vi "Build Qualified Class Private Data Name.vi"(1 "Qualified LabVIEW Class Name":string[](array[string])) -> (0 "Qualified LabVIEW Class Private Data Name":string)   [LabVIEW 2020]
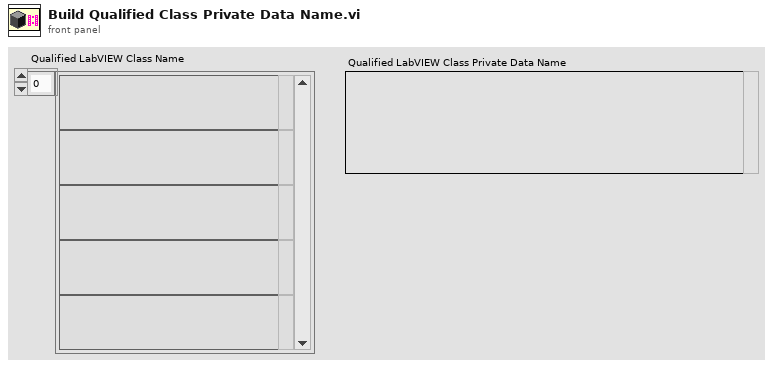
[diagram p1: front panel]
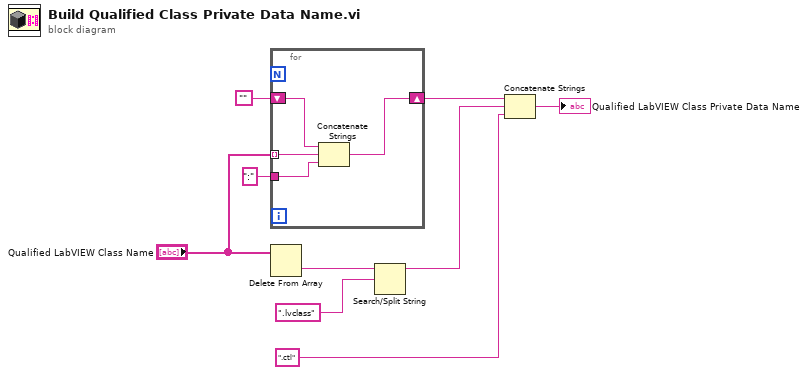
[diagram p0: block diagram]
diagram:
  n1 = for {
    tunnel: "Qualified LabVIEW Class Name" -> [w13] mode=indexing
    shift-right: [w12] -> w9
    shift-left: "" -> [w11]
    tunnel: ":" -> [w10]
    n2 = Concatenate Strings(w11, w13, w10) -> (w12:string)
  }
  n3 = Delete From Array(array="Qualified LabVIEW Class Name") -> (deleted portion=w4:string)  [unwired: 2 in, 1 out]
  n4 = Search/Split String(string=w4, search string/char (-)=".lvclass") -> (substring before match=w2:string)  [unwired: 1 in, 2 out]
  n5 = Concatenate Strings(w9, w2, ".ctl") -> (→"Qualified LabVIEW Class Private Data Name":string)
